vi "JV Measurement_Keithley 2400.vi"(9 "Max (V)":dbl, 11 "Step (V)":dbl=0.1) -> ()   [LabVIEW 2011]
uses:
  <vilib>/Utility/file.llb/Write To Spreadsheet File (string).vi
  <instrlib>/keithley_24xx/Keithley 24XX/Keithley 24XX.lvlib
panel:
  in  "Measurement Delay (ms)":dbl
  in  "Sample Name":string
  in  "Device Area (cm^2)":dbl=0.12
  out "XY Graph":cluster{dbl[], dbl[]}(graph)
  in  "Experiment Title":string
  in  "User Name":string
  in  "Stabilisation level \n(A or V depending on mode)":dbl=-1.6
  in  "Stabilisation time (ms)":dbl
  in  "Stabilisation mode":u16(ring) items=["Voltage", "Current"]
  in  "Max to min voltage sweep first?":bool
  in  "Min (V)":dbl=-1.6
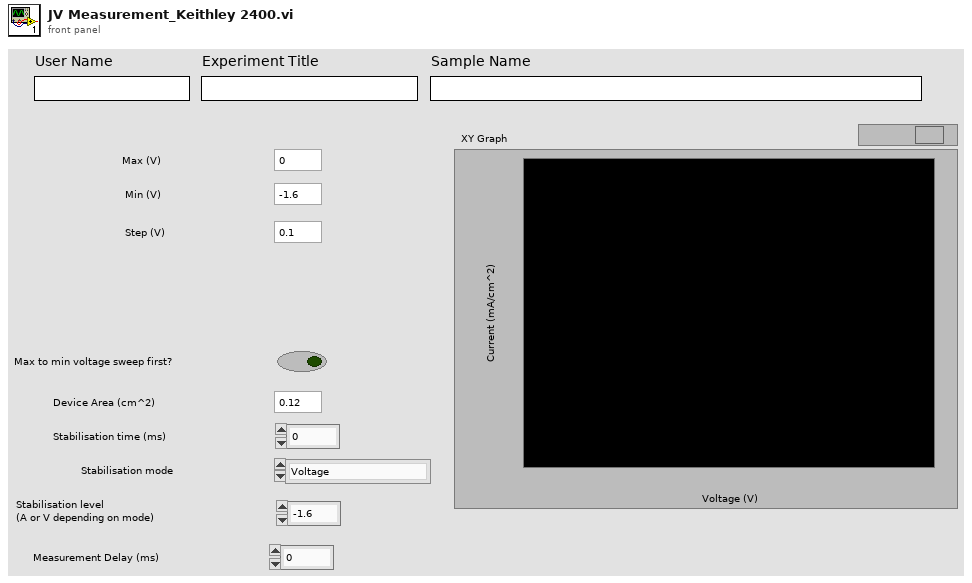
[diagram p1: front panel]
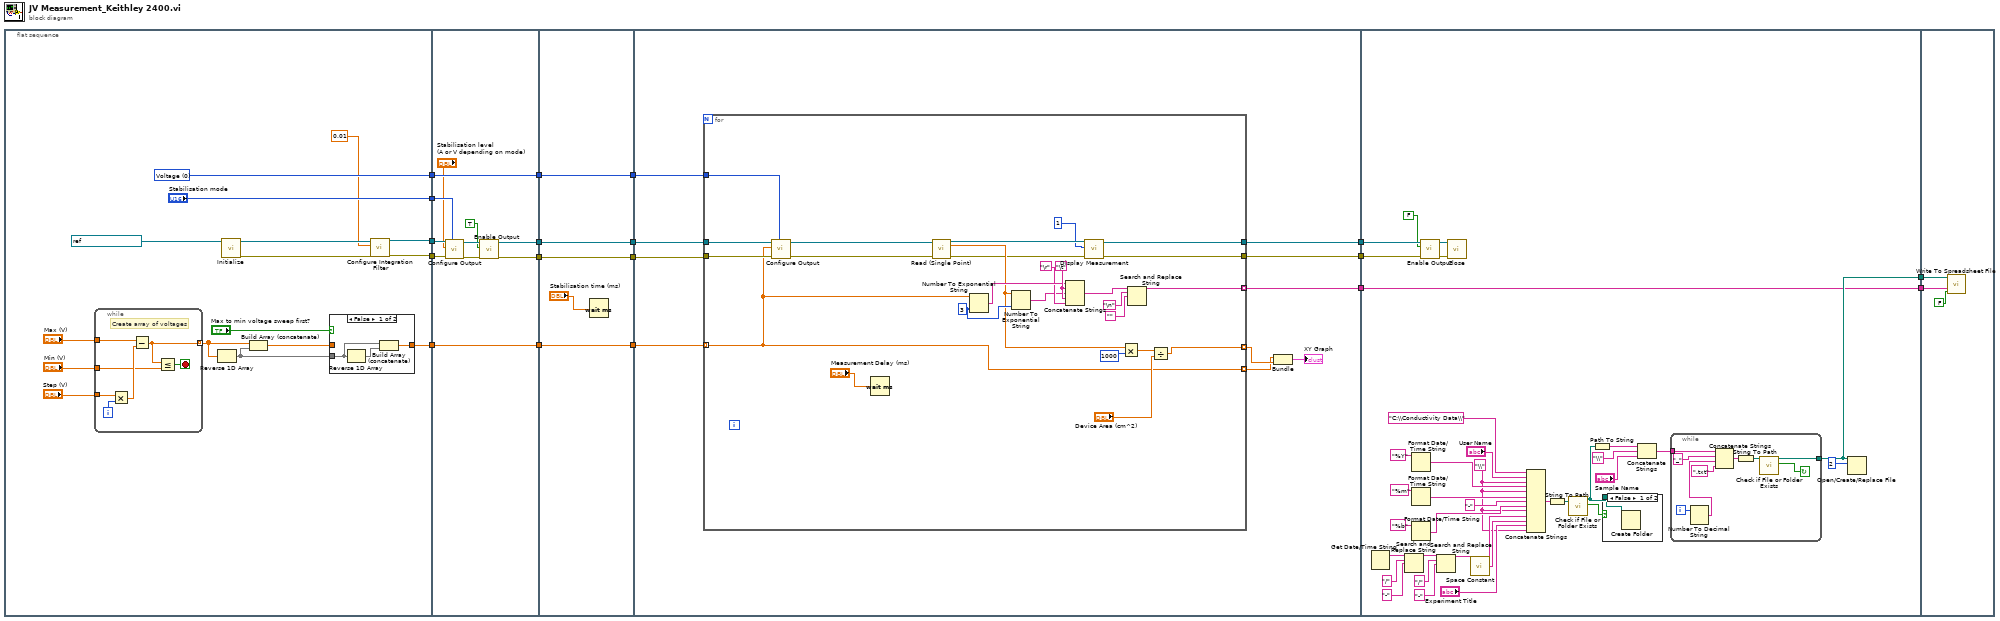
[diagram p0: block diagram]
diagram:
  n1 = flat-sequence {
    tunnel: [w25] -> w18
    tunnel: [w26] -> w17
    tunnel: ["Stabilisation mode"] -> w16
    tunnel: [w20] -> w15
    tunnel: [w21] -> w14
    tunnel: w18 -> [w48]
    tunnel: w17 -> [w56]
    tunnel: w16 -> [w49]
    tunnel: w15 -> [w52]
    tunnel: w14 -> [w53]
    tunnel: [w56] -> w13
    tunnel: [w51] -> w10
    tunnel: [w50] -> w8
    tunnel: [w48] -> w6
    tunnel: w13 -> [w61]
    tunnel: [w61] -> w12
    tunnel: [w60] -> w11
    tunnel: w10 -> [w60]
    tunnel: [w59] -> w9
    tunnel: w8 -> [w59]
    tunnel: [w57] -> w7
    tunnel: w6 -> [w57]
    tunnel: w12 -> [w69]
    tunnel: w11 -> [w71]
    tunnel: w9 -> [w70]
    tunnel: w7 -> [w68]
    tunnel: [w67] -> w5
    tunnel: [w66] -> w4
    tunnel: [w62] -> w1
    tunnel: w5 -> [w100]
    tunnel: w4 -> [w132]
    tunnel: [w101] -> w3
    tunnel: [w100] -> w2
    tunnel: w1 -> [w98]
    tunnel: w3 -> [w144]
    tunnel: w2 -> [w143]
    frame #0 {
      w25 = u16 0 items=["Voltage", "Current"] ("Source Function")
      n2 = while {
        tunnel: "Max (V)" -> [w45]
        tunnel: "Step (V)" -> [w44]
        tunnel: "Min (V)" -> [w41]
        tunnel: [w39] -> w27 mode=indexing
        i -> [w43]
        stop <- w40 stop-if-true
        # "Create array of voltages"
        n3 = Multiply(x=w44, y=w43) -> (x*y=w42:dbl)
        n4 = Subtract(x=w45, y=w42) -> (x-y=w39:dbl)
        n5 = Less Or Equal?(x=w39, y=w41) -> (x <= y?=w40:bool)
      }
      n6 = Reverse 1D Array(array=w27) -> (reversed array=w29:dbl[])
      n7 = call <instrlib>:"Initialize.vi"("VISA resource name"=refnum<visa-resource-name> "GPIB0::24::INSTR") -> ("error out"=w22:errorcluster, "VISA resource name out"=w23:refnum<visa-resource-name>)  [unwired: 4 in, 5 out]
      n8 = Build Array (concatenate)(w27, w29) -> (w30:dbl[])
      n9 = case shown="False" "Max to min voltage sweep first?" {
        tunnel: [w36 w38] -> w26
        tunnel: w30 -> [_ w38]
        tunnel: w29 -> [w37 _]
        frame False {
          n10 = Reverse 1D Array(array=w37) -> (reversed array=w35:dbl[])
          n11 = Build Array (concatenate)(w37, w35) -> (w36:dbl[])
        }
        frame True {
        }
      }
      n12 = call <instrlib>:"Configure Integration Filter.vi"("error in (no error)"=w22, "Measurement Speed (1 PLC)"=0.01, "VISA resource name"=w23) -> ("error out"=w20:errorcluster, "VISA resource name out"=w21:refnum<visa-resource-name>)  [unwired: 7 in]
    }
    frame #1 {
      n13 = call <instrlib>:"Configure Output.vi"("Source Mode  (0: Voltage)"=w49, "error in (no error)"=w52, "Output Level (0)"="Stabilisation level \n(A or V depending on mode)", "VISA resource name"=w53) -> ("error out"=w55:errorcluster, "VISA resource name out"=w54:refnum<visa-resource-name>)  [unwired: 6 in]
      n14 = call <instrlib>:"Enable Output.vi"("error in (no error)"=w55, "Enable Output (T: Enable)"=TRUE ("Output (Off)"), "VISA resource name"=w54) -> ("error out"=w50:errorcluster, "VISA resource name out"=w51:refnum<visa-resource-name>)  [unwired: 7 in]
    }
    frame #2 {
      n15 = Wait (ms)(milliseconds to wait="Stabilisation time (ms)") -> ()  [unwired: 1 out]
    }
    frame #3 {
      n16 = for {
        tunnel: w68 -> [w97]
        tunnel: w71 -> [w96]
        tunnel: w70 -> [w95]
        tunnel: [w73] -> w66
        tunnel: [w77] -> w63 mode=indexing
        tunnel: [w84] -> w64 mode=indexing
        tunnel: w69 -> [w77] mode=indexing
        tunnel: [w88] -> w67 mode=indexing
        tunnel: [w72] -> w62
        w79 = 3
        w92 = "\t"
        n17 = call <instrlib>:"Configure Output.vi"("Source Mode  (0: Voltage)"=w97, "error in (no error)"=w95, "Output Level (0)"=w77, "VISA resource name"=w96) -> ("error out"=w81:errorcluster, "VISA resource name out"=w82:refnum<visa-resource-name>)  [unwired: 6 in]
        n18 = Wait (ms)(milliseconds to wait="Measurement Delay (ms)") -> ()  [unwired: 1 out]
        n19 = call <instrlib>:"Read (Single Point).vi"("VISA resource name"=w82, "error in (no error)"=w81) -> ("VISA resource name out"=w76:refnum<visa-resource-name>, "Current"=w78:sgl, "error out"=w75:errorcluster)  [unwired: 7 in, 4 out]
        n20 = Number To Exponential String(number=w77, precision (6)=w79) -> (E-format string=w90:string)  [unwired: 2 in]
        n21 = Number To Exponential String(number=w78, precision (6)=w79) -> (E-format string=w80:string)  [unwired: 2 in]
        n22 = Concatenate Strings(w90, w92, w80, w92, "\r") -> (w94:string)
        n23 = call <instrlib>:"Display Measurement.vi"("error in (no error)"=w75, "Displayed Measurement (0: Voltage)"=1, "VISA resource name"=w76) -> ("error out"=w72:errorcluster, "VISA resource name out"=w73:refnum<visa-resource-name>)  [unwired: 7 in]
        n24 = Multiply(x=w78, y=1000) -> (x*y=w87:sgl)
        n25 = Search and Replace String(input string=w94, search string="\n", replace string="") -> (result string=w88:string)  [unwired: 5 in, 3 out]
        n26 = Divide(x=w87, y="Device Area (cm^2)") -> (x/y=w84:dbl)
      }
      n27 = Bundle(w63, w64) -> (→"XY Graph":cluster{dbl[], dbl[]})  [unwired: 1 in]
    }
    frame #4 {
      w111 = "\\"
      n28 = Get Date/Time String() -> (date string=w120:string)  [unwired: 3 in, 1 out]
      n29 = Search and Replace String(input string=w120, search string="/", replace string="-") -> (result string=w115:string)  [unwired: 5 in, 3 out]
      n30 = Format Date/Time String(time format string (%c)="%Y") -> (date/time string=w124:string)  [unwired: 2 in]
      n31 = Format Date/Time String(time format string (%c)="%m") -> (date/time string=w123:string)  [unwired: 2 in]
      n32 = Format Date/Time String(time format string (%c)="%b") -> (date/time string=w122:string)  [unwired: 2 in]
      n33 = call <instrlib>:"Enable Output.vi"("error in (no error)"=w98, "Enable Output (T: Enable)"=FALSE ("Output (Off)"), "VISA resource name"=w132) -> ("error out"=w130:errorcluster, "VISA resource name out"=w131:refnum<visa-resource-name>)  [unwired: 7 in]
      n34 = Search and Replace String(input string=w115, search string="/", replace string="-") -> (result string=w114:string)  [unwired: 5 in, 3 out]
      n35 = call <instrlib>:"Close.vi"("error in (no error)"=w130, "VISA resource name"=w131) -> ()  [unwired: 9 in, 1 out]
      n36 = call <vilib>:"Space Constant.vi"() -> ("String"=w113:string)
      n37 = Concatenate Strings("C:\\Conductivity Data\\", "User Name", w111, w124, w111, w123, "-", w122, w111, w114, w113, "Experiment Title", w111) -> (w104:string)
      n38 = String To Path(string=w104) -> (path=w103:path)
      n39 = call <vilib>:"Check if File or Folder Exists.vi"("path"=w103) -> ("file or folder exists?"=w107:bool, "dup path"=w109:path)  [unwired: 8 in, 1 out]
      n40 = Path To String(path=w109) -> (string=w108:string)
      n41 = case shown="False" w107 {
        tunnel: w109 -> [w133 _]
        frame False {
          n42 = Create Folder(path (use dialog)=w133) -> ()  [unwired: 2 in, 3 out]
        }
        frame True {
        }
      }
      n43 = Concatenate Strings(w108, "\\", "Sample Name") -> (w102:string)
      n44 = while {
        tunnel: w102 -> [w142]
        tunnel: [w134] -> w101
        i -> [w140]
        stop <- w135 continue-if-true
        n45 = Number To Decimal String(number=w140) -> (decimal integer string=w139:string)  [unwired: 1 in]
        n46 = Concatenate Strings(w142, "_", w139, ".txt") -> (w136:string)
        n47 = String To Path(string=w136) -> (path=w137:path)
        n48 = call <vilib>:"Check if File or Folder Exists.vi"("path"=w137) -> ("file or folder exists?"=w135:bool, "dup path"=w134:path)  [unwired: 8 in, 1 out]
      }
      n49 = Open/Create/Replace File(file path (use dialog)=w101, operation (0:open)=2) -> ()  [unwired: 4 in, 3 out]
    }
    frame #5 {
      n50 = call-poly <vilib>:"Write To Spreadsheet File.vi"("append to file? (new file:F)"=FALSE, "1D data"=w143, "file path (dialog if empty)"=w144) -> ()  [unwired: 5 in, 1 out]
    }
  }
